vi "EJERCICIO 1.vi"() -> ()   [LabVIEW 2014]
uses:
  RGB.ctl
panel:
  out "Array":bool[][](array[boolean])
  out "Umbralización":picture
  in  "Umbral":u8(slide) scale=0.0..255.0
  out "Escala de grises":picture
  in  "stop":bool
  in  "Enum":T1
  out "Rojo":picture
  out "Verde":picture
  out "Azul":picture
  out "new picture":picture
  in  "Path":path
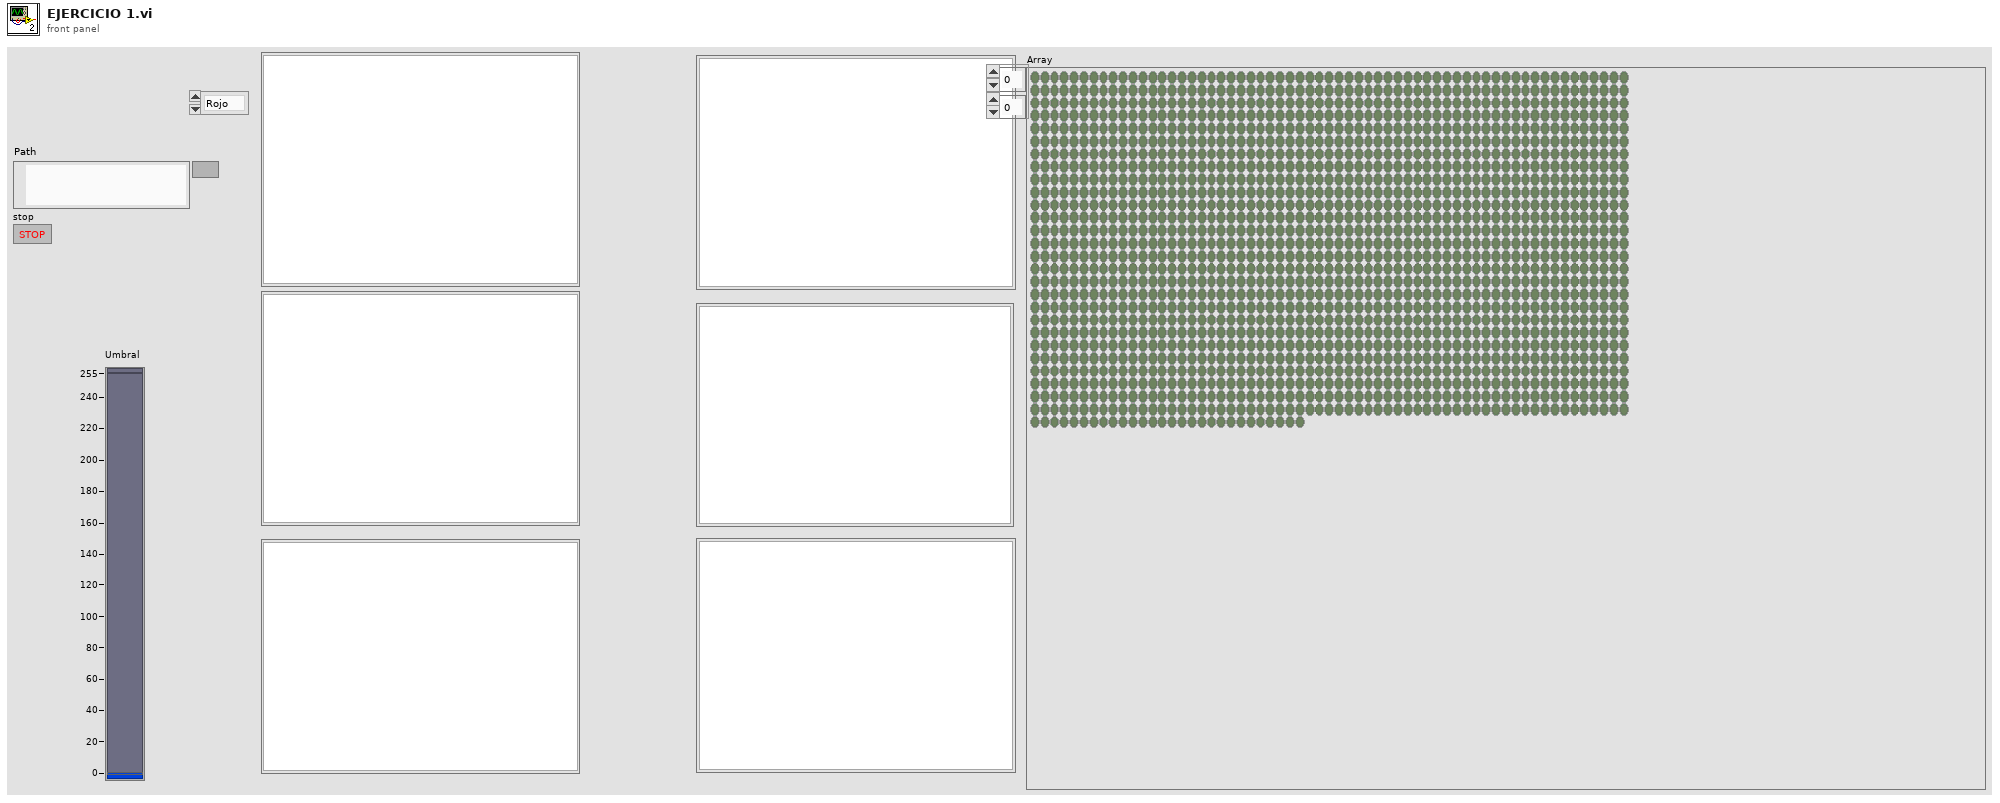
[diagram p1: front panel]
types:
  T1 = typedef "RGB.ctl" = enum16{"Rojo", "Verde", "Azul"}
  T2 = typedef "imagedata.ctl" = cluster{"image type":i32, "image depth":i32, "image":u8[], "mask":u8[], "colors":u32[], "Rectangle":cluster{"left":i16, "top":i16, "right":i16, "bottom":i16}}
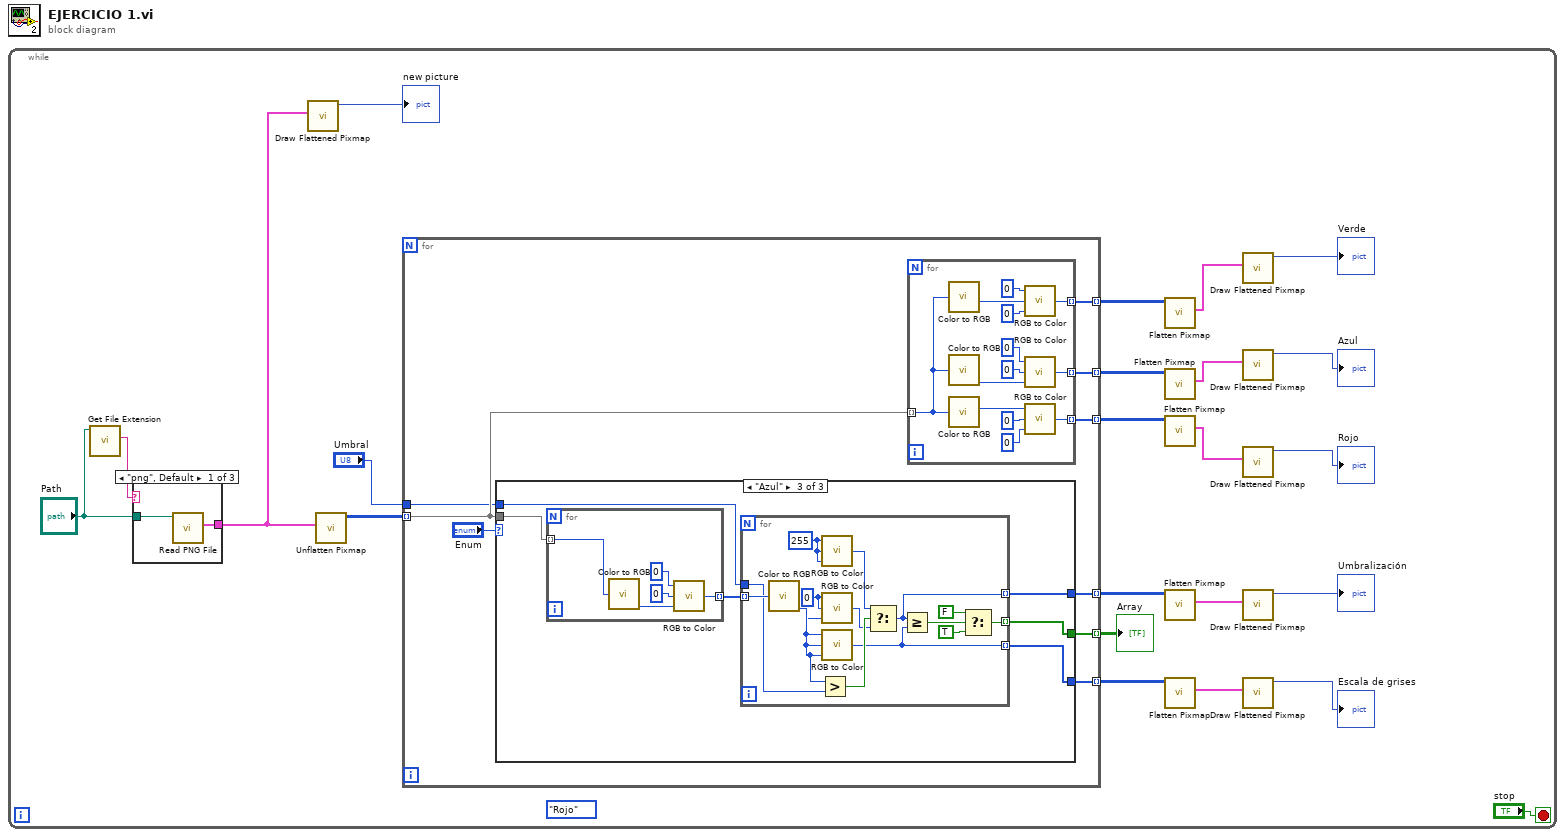
[diagram p0: block diagram]
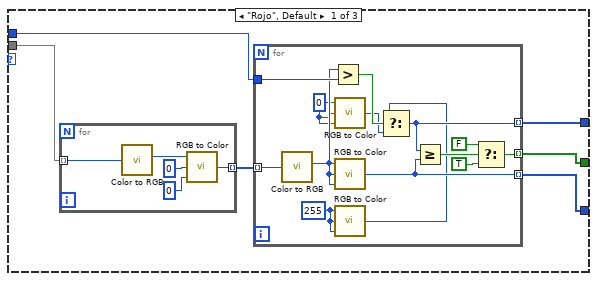
[diagram p2: hidden frame]
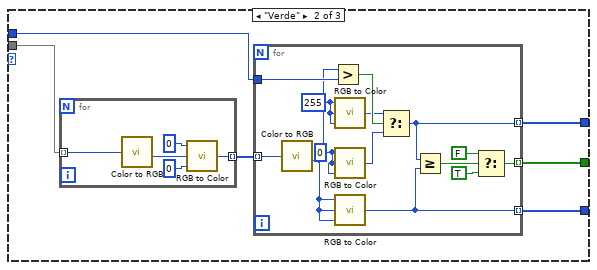
[diagram p3: hidden frame]
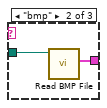
[diagram p4: hidden frame]
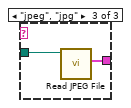
[diagram p5: hidden frame]
diagram:
  n1 = while {
    stop <- "stop" stop-if-true
    (unwired) RGB."Rojo"
    n2 = call <vilib>:"Get File Extension.vi"("file"="Path") -> ("lowercase file extension"=w22:string)  [unwired: 7 in, 3 out]
    n3 = case shown="\"png\", Default" w22 {
      tunnel: [w122 w124 w126] -> w20
      tunnel: "Path" -> [w121 w123 w125]
      frame "png", Default {
        n4 = call <vilib>:"Read PNG File.vi"("path to PNG file"=w121) -> ("image data"=w122:T2)  [unwired: 8 in, 2 out]
      }
      frame "bmp" {
        n5 = call <vilib>:"Read BMP File.vi"("path to BMP file"=w123) -> ("image data"=w124:T2)  [unwired: 8 in, 2 out]
      }
      frame "jpeg", "jpg" {
        n6 = call <vilib>:"Read JPEG File.vi"("path to JPEG file"=w125) -> ("image data"=w126:T2)  [unwired: 8 in, 2 out]
      }
    }
    n7 = call <vilib>:"Draw Flattened Pixmap.vi"("image data"=w20) -> ("new picture"=→"new picture":picture)  [unwired: 8 in]
    n8 = call <vilib>:"Unflatten Pixmap.vi"("image data"=w20) -> ("24-bit pixmap"=w9:u32[][])  [unwired: 4 in, 6 out]
    n9 = for {
      tunnel: w9 -> [w31] mode=indexing
      tunnel: [w32] -> w10 mode=indexing
      tunnel: [w29] -> w12 mode=indexing
      tunnel: [w28] -> w11 mode=indexing
      tunnel: [w27] -> w6 mode=indexing
      tunnel: [w26] -> w3 mode=indexing
      tunnel: [w25] -> w2 mode=indexing
      tunnel: "Umbral" -> [w24]
      n10 = case shown="\"Azul\"" "Enum" {
        tunnel: w31 -> [w38 w63 w88]
        tunnel: [w36 w61 w86] -> w27
        tunnel: [w35 w59 w84] -> w26
        tunnel: w24 -> [w34 w60 w85]
        tunnel: [w33 w58 w83] -> w25
        frame "Rojo", Default {
          n11 = for {
            tunnel: [w57] -> w37 mode=indexing
            tunnel: w38 -> [w56] mode=indexing
            n12 = call <vilib>:"Color to RGB.vi"("Color"=w56) -> ("R"=w55:u8)  [unwired: 3 out]
            n13 = call <vilib>:"RGB to Color.vi"("B"=u8 0, "G"=u8 0, "R"=w55) -> ("Color"=w57:u32)
          }
          n14 = for {
            tunnel: [w44] -> w36 mode=indexing
            tunnel: w37 -> [w52] mode=indexing
            tunnel: [w47] -> w35 mode=indexing
            tunnel: w34 -> [w50]
            tunnel: [w45] -> w33 mode=indexing
            w41 = u8 255 ("R")
            w42 = u8 0 ("R")
            n15 = call <vilib>:"Color to RGB.vi"("Color"=w52) -> ("R"=w43:u8)  [unwired: 3 out]
            n16 = Greater?(x=w43, y=w50) -> (0:w51:bool)
            n17 = call <vilib>:"RGB to Color.vi"("B"=w42, "G"=w42, "R"=w42) -> ("Color"=w40:u32)
            n18 = call <vilib>:"RGB to Color.vi"("B"=w43, "G"=w43, "R"=w43) -> ("Color"=w44:u32)
            n19 = call <vilib>:"RGB to Color.vi"("B"=w41, "G"=w41, "R"=w41) -> ("Color"=w39:u32)
            n20 = Select(t=w39, s=w51, f=w40) -> (s? t:f=w47:u32)
            n21 = Greater Or Equal?(x=w47, y=w44) -> (x >= y?=w46:bool)
            n22 = Select(t=FALSE, s=w46, f=TRUE) -> (s? t:f=w45:bool)
          }
        }
        frame "Verde" {
          n23 = for {
            tunnel: [w82] -> w62 mode=indexing
            tunnel: w63 -> [w81] mode=indexing
            n24 = call <vilib>:"Color to RGB.vi"("Color"=w81) -> ("G"=w80:u8)  [unwired: 3 out]
            n25 = call <vilib>:"RGB to Color.vi"("B"=u8 0, "G"=w80, "R"=u8 0) -> ("Color"=w82:u32)
          }
          n26 = for {
            tunnel: [w69] -> w61 mode=indexing
            tunnel: w62 -> [w77] mode=indexing
            tunnel: w60 -> [w75]
            tunnel: [w70] -> w59 mode=indexing
            tunnel: [w67] -> w58 mode=indexing
            w64 = u8 0 ("R")
            w65 = u8 255 ("R")
            n27 = call <vilib>:"Color to RGB.vi"("Color"=w77) -> ("G"=w66:u8)  [unwired: 3 out]
            n28 = Greater?(x=w66, y=w75) -> (0:w76:bool)
            n29 = call <vilib>:"RGB to Color.vi"("B"=w65, "G"=w65, "R"=w65) -> ("Color"=w74:u32)
            n30 = call <vilib>:"RGB to Color.vi"("B"=w64, "G"=w64, "R"=w64) -> ("Color"=w73:u32)
            n31 = call <vilib>:"RGB to Color.vi"("B"=w66, "G"=w66, "R"=w66) -> ("Color"=w69:u32)
            n32 = Select(t=w74, s=w76, f=w73) -> (s? t:f=w70:u32)
            n33 = Greater Or Equal?(x=w70, y=w69) -> (x >= y?=w68:bool)
            n34 = Select(t=FALSE, s=w68, f=TRUE) -> (s? t:f=w67:bool)
          }
        }
        frame "Azul" {
          n35 = for {
            tunnel: [w107] -> w87 mode=indexing
            tunnel: w88 -> [w106] mode=indexing
            n36 = call <vilib>:"Color to RGB.vi"("Color"=w106) -> ("B"=w105:u8)  [unwired: 3 out]
            n37 = call <vilib>:"RGB to Color.vi"("B"=w105, "G"=u8 0, "R"=u8 0) -> ("Color"=w107:u32)
          }
          n38 = for {
            tunnel: [w98] -> w86 mode=indexing
            tunnel: w87 -> [w102] mode=indexing
            tunnel: w85 -> [w100]
            tunnel: [w99] -> w84 mode=indexing
            tunnel: [w96] -> w83 mode=indexing
            w89 = u8 0 ("R")
            w90 = u8 255 ("R")
            n39 = call <vilib>:"Color to RGB.vi"("Color"=w102) -> ("B"=w93:u8)  [unwired: 3 out]
            n40 = Greater?(x=w93, y=w100) -> (0:w101:bool)
            n41 = call <vilib>:"RGB to Color.vi"("B"=w90, "G"=w90, "R"=w90) -> ("Color"=w91:u32)
            n42 = call <vilib>:"RGB to Color.vi"("B"=w89, "G"=w89, "R"=w89) -> ("Color"=w92:u32)
            n43 = call <vilib>:"RGB to Color.vi"("B"=w93, "G"=w93, "R"=w93) -> ("Color"=w98:u32)
            n44 = Select(t=w91, s=w101, f=w92) -> (s? t:f=w99:u32)
            n45 = Greater Or Equal?(x=w99, y=w98) -> (x >= y?=w97:bool)
            n46 = Select(t=FALSE, s=w97, f=TRUE) -> (s? t:f=w96:bool)
          }
        }
      }
      n47 = for {
        tunnel: w31 -> [w109] mode=indexing
        tunnel: [w120] -> w32 mode=indexing
        tunnel: [w111] -> w29 mode=indexing
        tunnel: [w110] -> w28 mode=indexing
        n48 = call <vilib>:"Color to RGB.vi"("Color"=w109) -> ("G"=w115:u8)  [unwired: 3 out]
        n49 = call <vilib>:"Color to RGB.vi"("Color"=w109) -> ("B"=w118:u8)  [unwired: 3 out]
        n50 = call <vilib>:"Color to RGB.vi"("Color"=w109) -> ("R"=w108:u8)  [unwired: 3 out]
        n51 = call <vilib>:"RGB to Color.vi"("B"=u8 0, "G"=w115, "R"=u8 0 ("G")) -> ("Color"=w111:u32)
        n52 = call <vilib>:"RGB to Color.vi"("B"=w118, "G"=u8 0, "R"=u8 0 ("B")) -> ("Color"=w120:u32)
        n53 = call <vilib>:"RGB to Color.vi"("B"=u8 0, "G"=u8 0, "R"=w108) -> ("Color"=w110:u32)
      }
    }
    "Array" <- w2
    n54 = call <vilib>:"Flatten Pixmap.vi"("24-bit pixmap"=w12) -> ("image data"=w17:T2)  [unwired: 10 in]
    n55 = call <vilib>:"Flatten Pixmap.vi"("24-bit pixmap"=w10) -> ("image data"=w18:T2)  [unwired: 10 in]
    n56 = call <vilib>:"Flatten Pixmap.vi"("24-bit pixmap"=w11) -> ("image data"=w14:T2)  [unwired: 10 in]
    n57 = call <vilib>:"Flatten Pixmap.vi"("24-bit pixmap"=w3) -> ("image data"=w5:T2)  [unwired: 10 in]
    n58 = call <vilib>:"Flatten Pixmap.vi"("24-bit pixmap"=w6) -> ("image data"=w7:T2)  [unwired: 10 in]
    n59 = call <vilib>:"Draw Flattened Pixmap.vi"("image data"=w17) -> ("new picture"=→"Verde":picture)  [unwired: 8 in]
    n60 = call <vilib>:"Draw Flattened Pixmap.vi"("image data"=w18) -> ("new picture"=→"Azul":picture)  [unwired: 8 in]
    n61 = call <vilib>:"Draw Flattened Pixmap.vi"("image data"=w14) -> ("new picture"=→"Rojo":picture)  [unwired: 8 in]
    n62 = call <vilib>:"Draw Flattened Pixmap.vi"("image data"=w5) -> ("new picture"=→"Umbralización":picture)  [unwired: 8 in]
    n63 = call <vilib>:"Draw Flattened Pixmap.vi"("image data"=w7) -> ("new picture"=→"Escala de grises":picture)  [unwired: 8 in]
  }
